vi "StopMotor.vi"(8 "error in (no error)":errorcluster, 11 "ThorlabsLabJack in":refnum<class "ThorlabsLabJack.lvclass">) -> (0 "error out":errorcluster, 3 "ThorlabsLabJack out":refnum<class "ThorlabsLabJack.lvclass">)   [LabVIEW 2018, in "ThorlabsLabJack.lvlib" / "ThorlabsLabJack.lvclass"]
uses:
  ThorlabsLabJack.lvclass
  ThorlabsLabJack.lvclass/ThorlabsLabJack.ctl
  C:/Projects/LabVIEW/In-Progress/Chetan Malpure/Axis/Thorlabs LabJack/Drivers/Thorlabs.MotionControl.IntegratedStepperMotorsCLI.dll
  Drivers/Thorlabs.MotionControl.IntegratedStepperMotorsCLI.dll
  91b5fc19-c8fb-4e29-ae9f-d63fcf16b306.vi
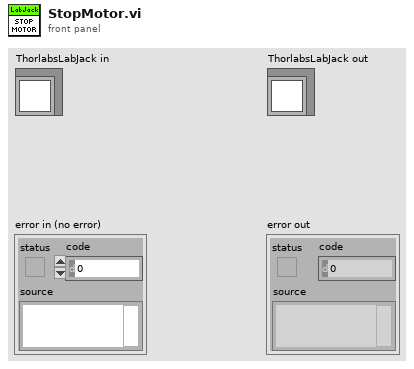
[diagram p1: front panel]
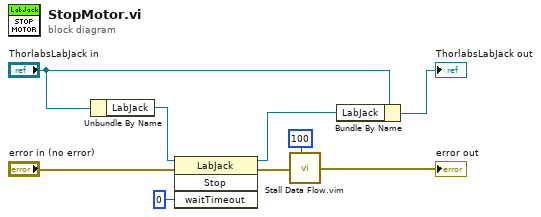
[diagram p0: block diagram]
diagram:
  n1 = Unbundle By Name("ThorlabsLabJack in") -> ("LabJack"=w8:refnum<k24>)
  n2 = invoke class="LabJack" method="Stop"(reference=w8, error in="error in (no error)", "waitTimeout"=0) -> (reference out=w4:refnum<k24>, error out=w6:errorcluster)  [unwired: 1 in, 2 out]
  n3 = call "Stall Data Flow.vim"("value in"=w6, "milliseconds to wait"=u32 100) -> ("value out"=→"error out":errorcluster)  [unwired: 1 out]
  n4 = Bundle By Name(cluster="ThorlabsLabJack in", "LabJack"=w4) -> (→"ThorlabsLabJack out":refnum<class "ThorlabsLabJack.lvclass">)
